vi "Handle Error.vi"(8 "error in (no error)":errorcluster, 11 "UDP_Service in":refnum<class "UDP_Service.lvclass">) -> (0 "error out":errorcluster, 2 "stop actor?":bool=TRUE, 3 "UDP_Service out":refnum<class "UDP_Service.lvclass">)   [LabVIEW 2016, in "CoreAssertAPI.lvlib" / "UDP_Service.lvclass"]
doc: "(<B>Filename</B>: Actor Framework.lvlib:Actor.lvclass:Handle Error.vi)\n\nDefines how the actor handles an error that occurred while processing a message. By default, this method does nothing except stop the actor."
uses:
  UDP_Service.lvclass
  <vilib>/ActorFramework/Actor/Actor.lvclass
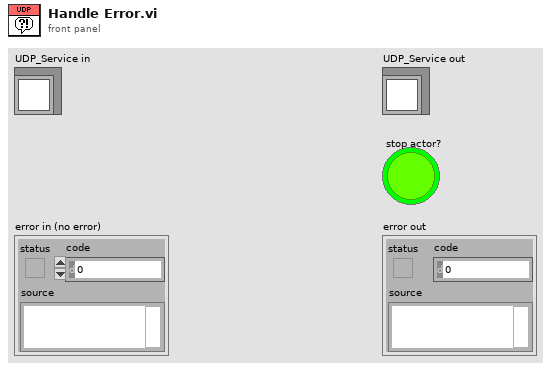
[diagram p1: front panel]
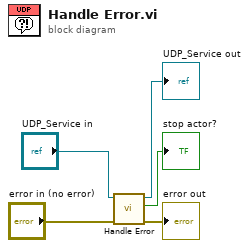
[diagram p0: block diagram]
diagram:
  n1 = call-parent "Handle Error.vi"("error in (no error)"="error in (no error)", "Actor in"="UDP_Service in") -> ("error out"=→"error out":errorcluster, "stop actor?"=→"stop actor?":bool, "Actor out"=→"UDP_Service out":refnum<class "UDP_Service.lvclass">)  [unwired: 7 in]
